vi "MultipleChannelEditorUI.vi"(8 "error in":errorcluster, 11 "cRIO repo in":refnum<class "_cRIORepo.lvclass">) -> (0 "error out":errorcluster, 3 "cRIO repo out":refnum<class "_cRIORepo.lvclass">)   [LabVIEW 2013, in "_cRIORepo.lvclass"]
uses:
  _cRIORepo.lvclass
  _cRIORepo.lvclass/_cRIORepo.ctl
panel:
  in  "Table":string[][](table)
  in  "Cancel":bool
  in  "OK":bool
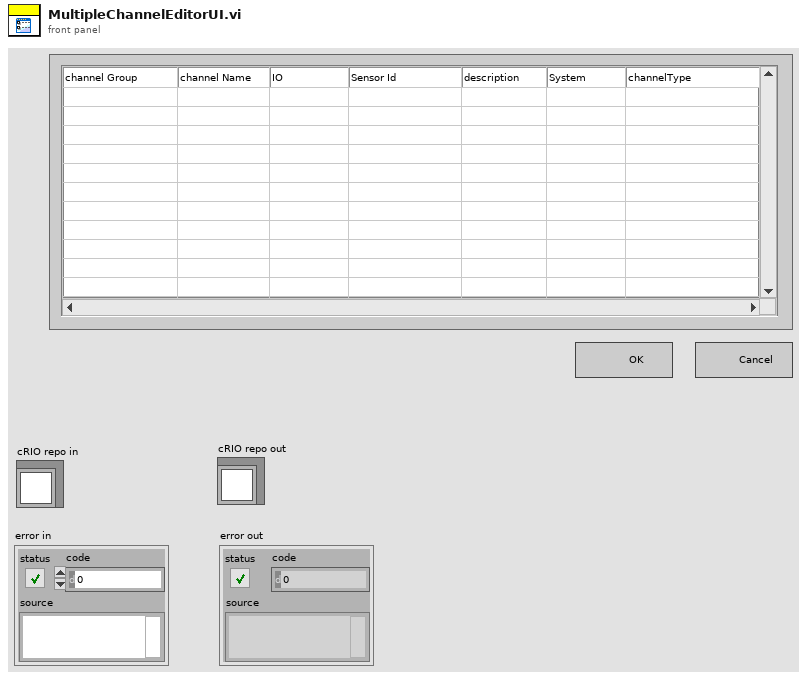
[diagram p1: front panel]
types:
  T1 = enum32{"Invalid", "Standard", "Closed", "Hidden", "Minimized", "Maximized"}
  T2 = typedef "_cRIORepo.lvclass/ChannelData.ctl" = cluster{"channel group":string, "channel name":string, "IO ":string, "sensor ID":string, "description":string, "system":string, "channel type":string}
  T3 = cluster{"Table[0]":string, "Table[1]":string, "Table[2]":string, "Table[3]":string, "Table[4]":string, "Table[5]":string, "Table[6]":string}
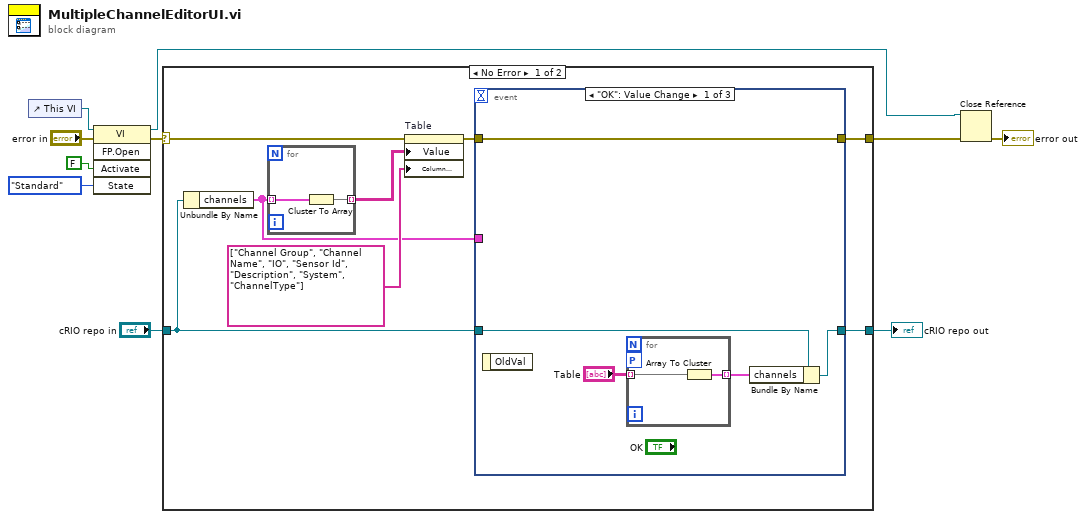
[diagram p0: block diagram]
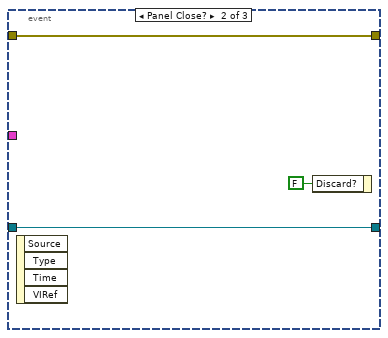
[diagram p2: hidden frame]
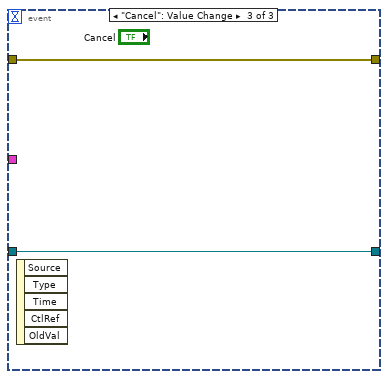
[diagram p3: hidden frame]
diagram:
  n1 = control-ref of="This VI"() -> (w7:refnum<vi>)
  n2 = invoke class="VI" method="FP.Open"(reference=w7, error in="error in", "Activate"=FALSE ("Activate?"), "State"=T1."Standard") -> (reference out=w2:refnum<vi>, error out=w3:errorcluster)  [unwired: 1 in, 3 out]
  n3 = case shown="No Error" w3 {
    selector: w3 -> [w18 w34]
    tunnel: "cRIO repo in" -> [w12 w33]
    tunnel: [w11 w33] -> w9
    tunnel: [w17 w34] -> w1
    frame No Error {
      n4 = Unbundle By Name(w12) -> ("channels"=w13:T2[])
      n5 = for {
        tunnel: w13 -> [w20] mode=indexing
        tunnel: [w19] -> w16 mode=indexing
        n6 = Cluster To Array(cluster=w20) -> (array=w19:string[])
      }
      n7 = property on="Table" class="Tbl (strict)"(error in=w18, "Value"=w16, "Column Headers[]"=string[] ["Channel Group", "Channel Name", "IO", "Sensor Id", "Description", "System", "ChannelType"] ("Column Header Strings[]")) -> (error out=w15:errorcluster)  [unwired: 1 in, 1 out]
      n8 = event shown="[0] \"OK\": Value Change" {
        selector: _ -> [_ _ _]
        dyn-events: _ -> [_ _ _]
        timeout: _ -> [_ _ _]
        tunnel: w15 -> [w25 w29 w31]
        tunnel: [w25 w29 w31] -> w17
        tunnel: w13 -> [_ _ _]
        tunnel: w12 -> [w23 w28 w32]
        tunnel: [w22 w28 w32] -> w11
        event "OK": Value Change {
          n9 = event-data() -> ()  [unwired: 1 in, 1 out]
          n10 = for {
            tunnel: "Table" -> [w27] mode=indexing
            tunnel: [w26] -> w21 mode=indexing
            workers-P: _ -> [_]
            n11 = Array To Cluster(array=w27) -> (cluster=w26:T3)
          }
          n12 = Bundle By Name(cluster=w23, "channels"=w21) -> (w22:refnum<class "_cRIORepo.lvclass">)
        }
        event Panel Close? {
          n13 = event-data() -> ()  [unwired: 1 in, 4 out]
          n14 = event-data("Discard?"=FALSE) -> ()  [unwired: 1 in, 1 out]
        }
        event "Cancel": Value Change {
          n15 = event-data() -> ()  [unwired: 1 in, 5 out]
        }
      }
    }
    frame Error {
    }
  }
  "cRIO repo out" <- w9
  n16 = Close Reference(reference=w2, error in (no error)=w1) -> (error out=→"error out":errorcluster)
